vi "Calc and Send Vector.vi"(8 "error in (no error)":errorcluster, 11 "RDS Mission Controller Actor in":refnum<class "RDS Mission Controller Actor.lvclass">) -> (0 "error out":errorcluster, 3 "RDS Mission Controller Actor out":refnum<class "RDS Mission Controller Actor.lvclass">)   [LabVIEW 2015, in "RDS Mission Controller Actor.lvlib" / "RDS Mission Controller Actor.lvclass"]
uses:
  RDS Mission Controller Actor.lvclass
  Libraries/RDS Child Messages/Helm/Heading Command/Heading Command Cntrl.ctl
  RDS Mission Controller Actor.lvclass/RDS Mission Controller Actor.ctl
  Libraries/Geo/RDS Libraries.lvlib
  Actors/RDS Helm Actor/RDS Helm Actor.lvlib
  Libraries/RDS Child Messages/RDS Child Messages.lvlib
  Actors/RDS Parent Actor/RDS Parent Actor/RDS Parent Actor.lvclass
panel:
  out "Bearing to Destination":dbl
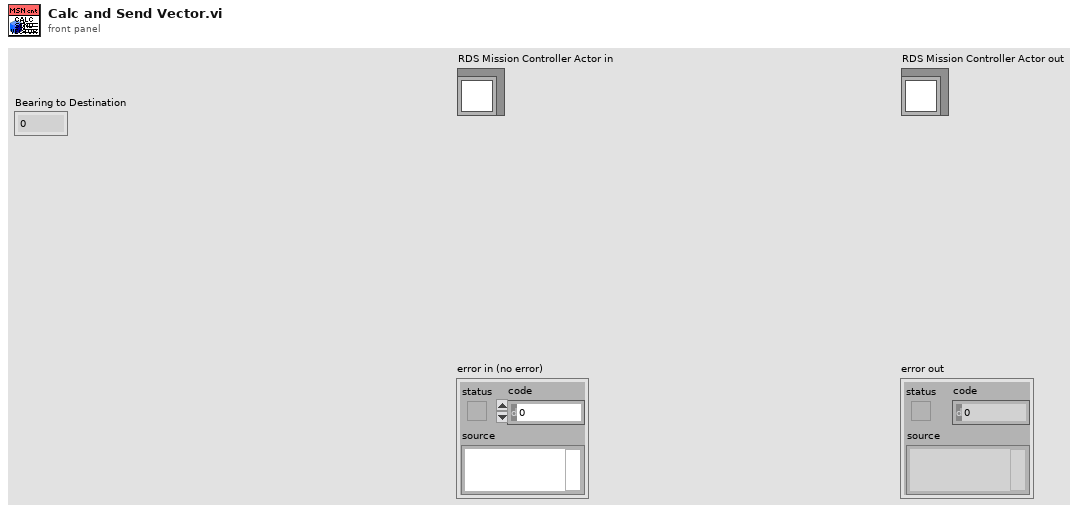
[diagram p1: front panel]
types:
  T1 = typedef "RDS Child Messages.lvlib/Heading Command Cntrl.ctl" = cluster{"Throttle":i16, "Heading":sgl, "Duration (s)":i16}
  T2 = typedef "RDS Mission Controller Actor.lvlib/MissionOp.ctl" = cluster{"MissionOp Type":enum16{"Waypoint", "Loiter", "Wait", "Deploy AIP", "Stow AIP"}, "Duration (s)":u16, "Throttle":i16, "GPS Latitude":dbl, "GPS Longitude":dbl, "Loiter Range (m)":u16}
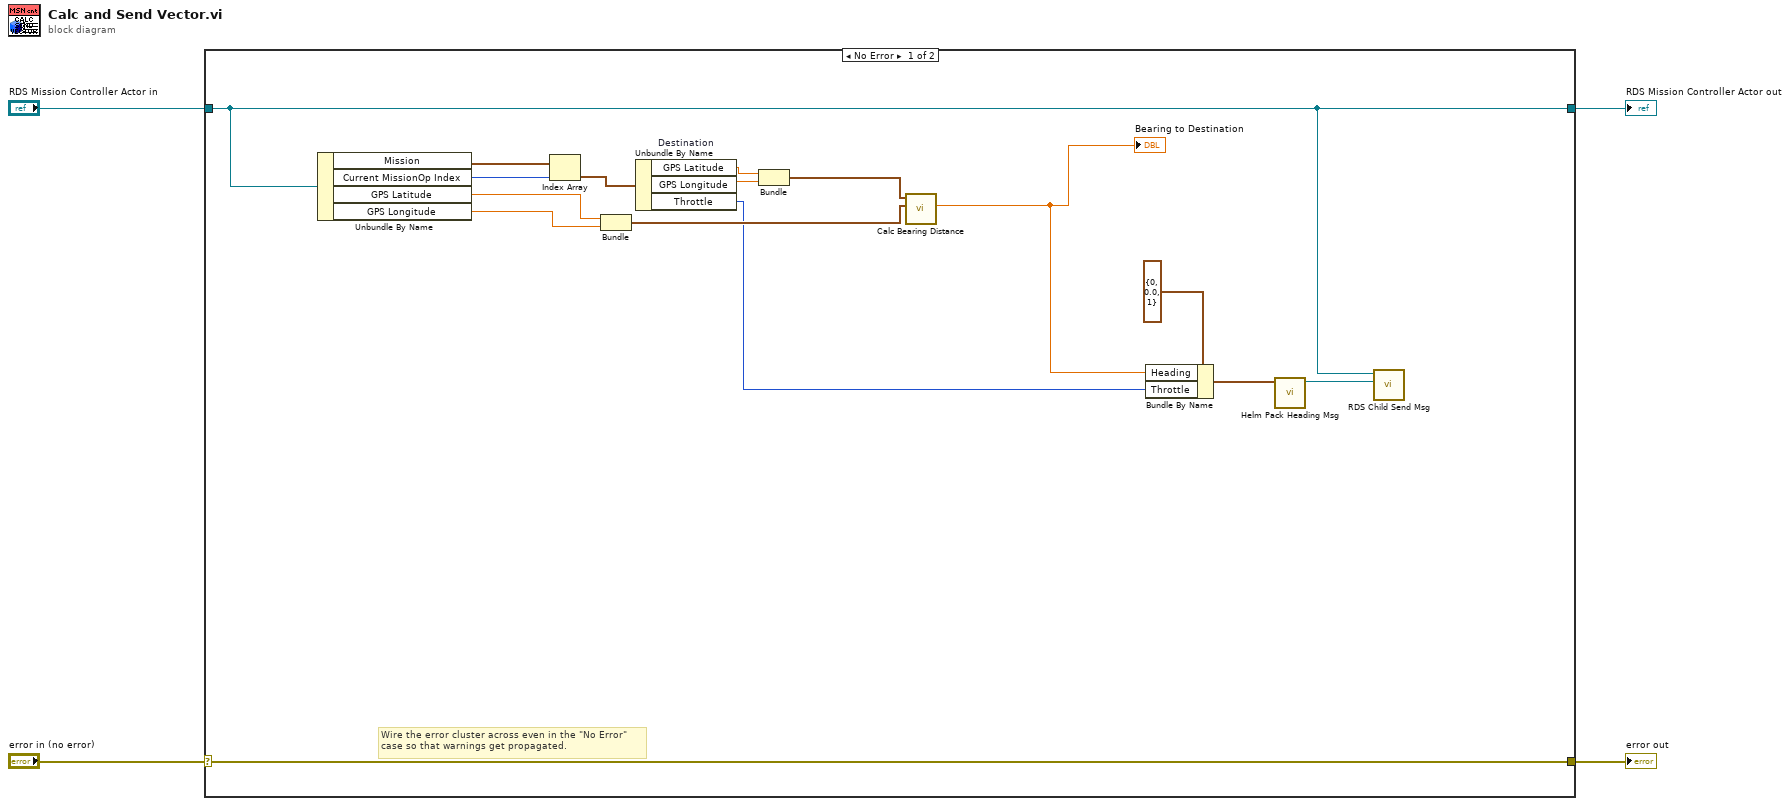
[diagram p0: block diagram]
diagram:
  n1 = case shown="No Error" "error in (no error)" {
    selector: "error in (no error)" -> [w20 w22]
    tunnel: [w20 w22] -> w2
    tunnel: [w5 w21] -> w1
    tunnel: "RDS Mission Controller Actor in" -> [w5 w21]
    frame No Error {
      # "Wire the error cluster across even in the \"No Error\"\ncase so that warnings get propagated."
      n2 = Unbundle By Name(w5) -> ("Mission"=w19:T2[], "Current MissionOp Index"=w18:i32, "GPS Latitude"=w13:ext, "GPS Longitude"=w12:ext)
      n3 = Index Array(array=w19, index=w18) -> (element=w17:T2)
      n4 = Bundle("GPS Latitude"=w13, "GPS Longitude"=w12) -> (w11:cluster{"GPS Latitude":ext, "GPS Longitude":ext})  [unwired: 1 in]
      n5 = Unbundle By Name "Destination"(w17) -> ("GPS Latitude"=w16:dbl, "GPS Longitude"=w15:dbl, "Throttle"=w7:i16)
      n6 = Bundle("GPS Latitude"=w16, "GPS Longitude"=w15) -> (w14:cluster{"GPS Latitude":dbl, "GPS Longitude":dbl})  [unwired: 1 in]
      n7 = call "Calc Bearing Distance.vi"("Current Location"=w11, "Destination"=w14) -> ("Bearing to Destination"=w8:dbl)  [unwired: 8 in, 1 out]
      "Bearing to Destination" <- w8
      n8 = Bundle By Name(cluster=T1 {"Throttle"=0, "Heading"=0.0, "Duration (s)"=1} ("Heading Command Control"), "Heading"=w8, "Throttle"=w7) -> (w9:T1)
      n9 = call "Helm Pack Heading Msg.vi"("Heading Command Control"=w9) -> ("Heading Command Msg out"=w6:refnum<class "Heading Command Msg.lvclass">)  [unwired: 9 in, 1 out]
      n10 = call "RDS Child Send Msg.vi"("RDS Message"=w6, "RDS Parent Actor in"=w5) -> ()  [unwired: 8 in, 2 out]
    }
    frame Error {
    }
  }
  "error out" <- w2
  "RDS Mission Controller Actor out" <- w1
